vi "DbRoomClusterToRoom.vi"(8 "error in":errorcluster, 10 "RoomTableCluster":T1 {"Flag3" min=0 max=1; "Flag2" min=0 max=1; "Flag1" min=0 max=1; "Flag0" min=0 max=1; "BedVacant" min=0 max=1}) -> (0 "error out":errorcluster, 2 "EventTime":timestamp, 3 "Room out":refnum<class "Room.lvclass">)   [LabVIEW 2015, in "DatabaseApi.lvlib"]
uses:
  DatabaseApi.lvlib
  TypeDef/Room/RoomTableCluster.ctl
  LVClasses/Room/Room.lvclass
  LVClasses/Room/Room.lvclass/Room.ctl
  LVClasses/Room/Write Flags.lvclass.vi
  LVClasses/Room/Write BedVacant.vi
  LVClasses/Room/Write Room Number.vi
  LVClasses/Room/Write InRoomPersonnel.vi
  LVClasses/Flags/Flags.lvclass
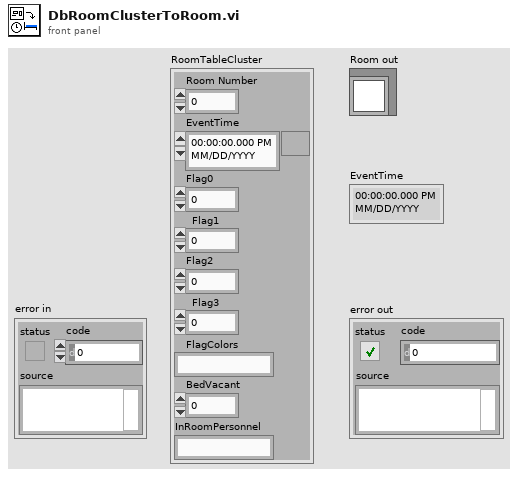
[diagram p1: front panel]
types:
  T1 = typedef "DatabaseApi.lvlib/RoomTableCluster.ctl" = cluster{"Room Number":i32, "EventTime":timestamp, "Flag0":i32, "Flag1":i32, "Flag2":i32, "Flag3":i32, "FlagColors":string, "BedVacant":i32, "InRoomPersonnel":string}
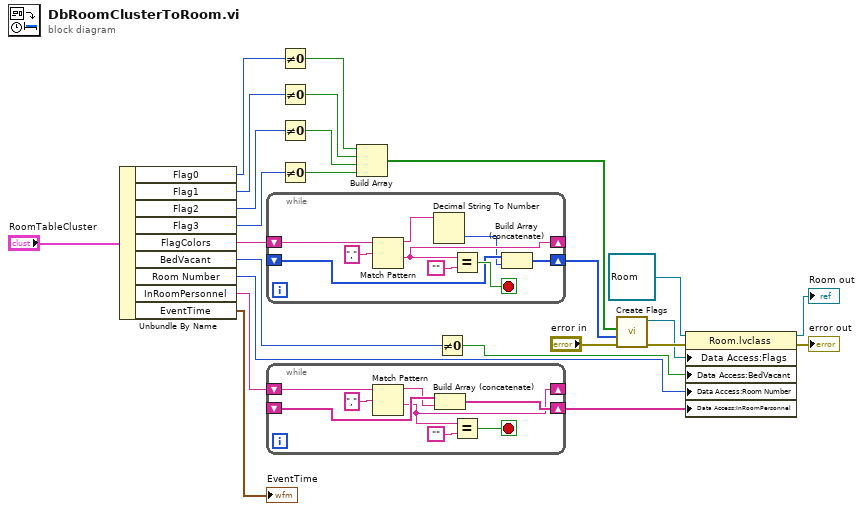
[diagram p0: block diagram]
diagram:
  n1 = Unbundle By Name("RoomTableCluster") -> ("Flag0"=w4:i32, "Flag1"=w3:i32, "Flag2"=w2:i32, "Flag3"=w1:i32, "FlagColors"=w11:string, "BedVacant"=w20:i32, "Room Number"=w19:i32, "InRoomPersonnel"=w17:string, "EventTime"=→"EventTime":timestamp)
  n2 = while {
    shift-right: [w31] -> w10
    shift-left: _ -> [w30]
    shift-right: [w27] -> _
    shift-left: w11 -> [w28]
    stop <- w33 stop-if-true
    n3 = Match Pattern(string=w28, regular expression="," ("search string/char (-)")) -> (before substring=w25:string, after substring=w27:string)  [unwired: 1 in, 2 out]
    n4 = Decimal String To Number(string=w25) -> (number=w26:i32)  [unwired: 2 in, 1 out]
    n5 = Equal?(x=w27, y="") -> (x = y?=w33:bool)
    n6 = Build Array (concatenate)(w30, w26) -> (w31:i32[])
  }
  n7 = while {
    shift-right: [w39] -> w18
    shift-left: _ -> [w38]
    shift-right: [w34] -> _
    shift-left: w17 -> [w36]
    stop <- w41 stop-if-true
    n8 = Match Pattern(string=w36, regular expression="," ("search string/char (-)")) -> (before substring=w35:string, after substring=w34:string)  [unwired: 1 in, 2 out]
    n9 = Build Array (concatenate)(w38, w35) -> (w39:string[])
    n10 = Equal?(x=w34, y="") -> (x = y?=w41:bool)
  }
  n11 = Not Equal To 0?(x=w4) -> (x != 0?=w8:bool)
  n12 = Not Equal To 0?(x=w3) -> (x != 0?=w6:bool)
  n13 = Not Equal To 0?(x=w2) -> (x != 0?=w5:bool)
  n14 = Not Equal To 0?(x=w1) -> (x != 0?=w9:bool)
  n15 = Build Array(w8, w6, w5, w9) -> (w7:bool[])
  n16 = Not Equal To 0?(x=w20) -> (x != 0?=w23:bool)
  n17 = call "Create Flags.vi"("error in"="error in", "Color"=w10, "State"=w7) -> ("error out"=w22:errorcluster, "reference out"=w21:refnum<class "Flags.lvclass">)  [unwired: 7 in]
  n18 = property class="Room.lvclass"(reference=refnum<class "Room.lvclass"> refnum ("Room.lvclass"), error in=w22, "Data Access:Flags"=w21, "Data Access:BedVacant"=w23, "Data Access:Room Number"=w19, "Data Access:InRoomPersonnel"=w18) -> (reference out=→"Room out":refnum<class "Room.lvclass">, error out=→"error out":errorcluster)
